vi "WPI_GyroConstants.vi"() -> (0 "Deadband":dbl, 1 "Samples Per Second":dbl=50.0, 2 "Averaging Bits":u8, 3 "Oversample Bits":u8=10, 5 "Gain (VoltsPerDegreePerSecond)":dbl=0.007)   [LabVIEW 2017]
doc: "This software is licensed. Open the labview\\readme\\WPI Robotics Library Open Source License.txt file for more information."
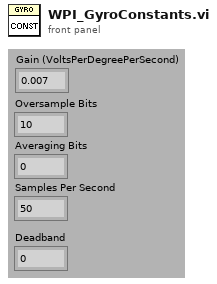
[diagram p1: front panel]
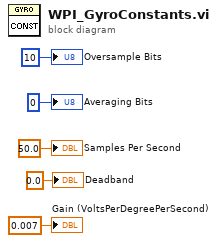
[diagram p0: block diagram]
diagram:
  "Oversample Bits" <- u8 10 ("Oversample Bits")
  "Averaging Bits" <- u8 0 ("Oversample Bits")
  "Samples Per Second" <- 50.0 ("Oversample Bits")
  "Deadband" <- 0.0 ("Deadband")
  "Gain (VoltsPerDegreePerSecond)" <- 0.007 ("VoltsPerDegreePerSecond")
